vi "CalculatePhaseMagnitude_5761.vi"(7 "Max num channels":i32, 8 "unwrap phase":bool, 9 "phase reference channel":i32, 10 "previous phase":dbl[](array[numeric]), 11 "data":dbl[][](array[numeric])) -> (1 "last phase":dbl[](array[numeric]), 2 "Magnitude":dbl[][](array[numeric]), 3 "Phase":dbl[][](array[numeric]))   [LabVIEW 2018, in "Scope5782_six_channel.lvclass"]
uses:
  Scope5782_six_channel.lvclass
  <vilib>/Analysis/coordinate.llb/Angle Units.ctl
  <vilib>/Analysis/NI_AALPro.lvlib
  <vilib>/Analysis/NI_AAL_Angle.lvlib
panel:
  in  "Max num channels 2":i32
  # "each row is I and then Q of one channel"
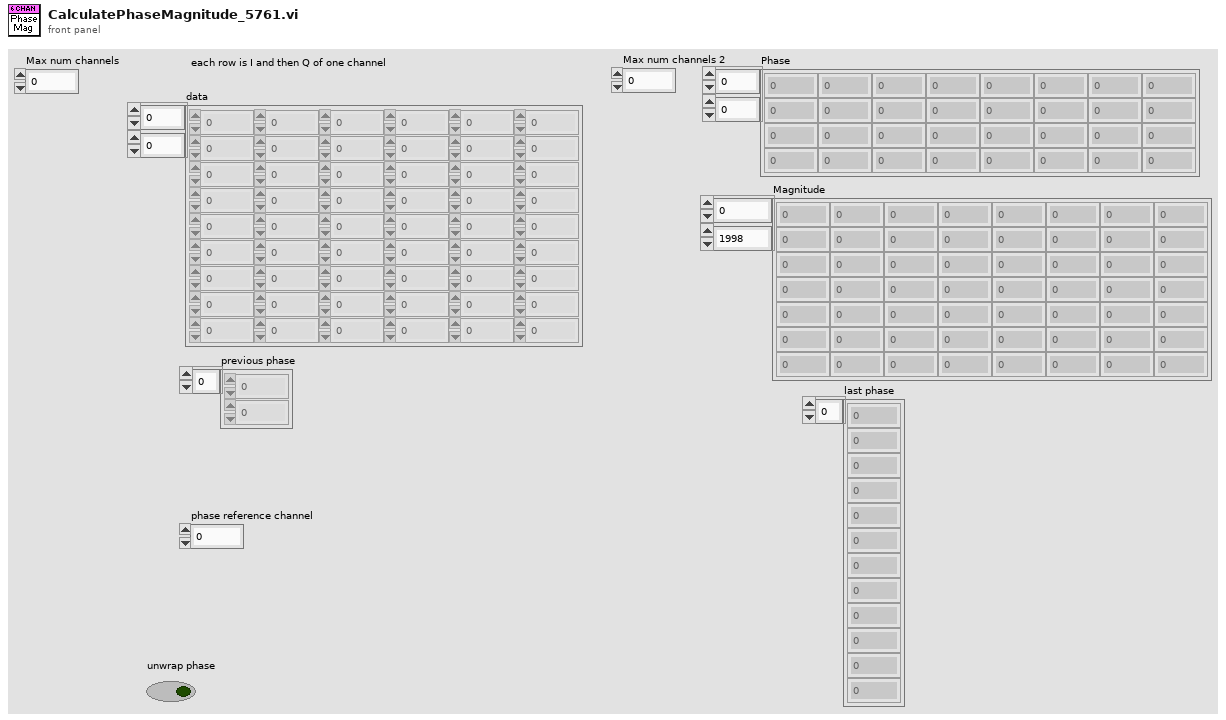
[diagram p1: front panel]
types:
  T1 = typedef "NI_AAL_Angle.lvlib/Angle Units.ctl" = i32
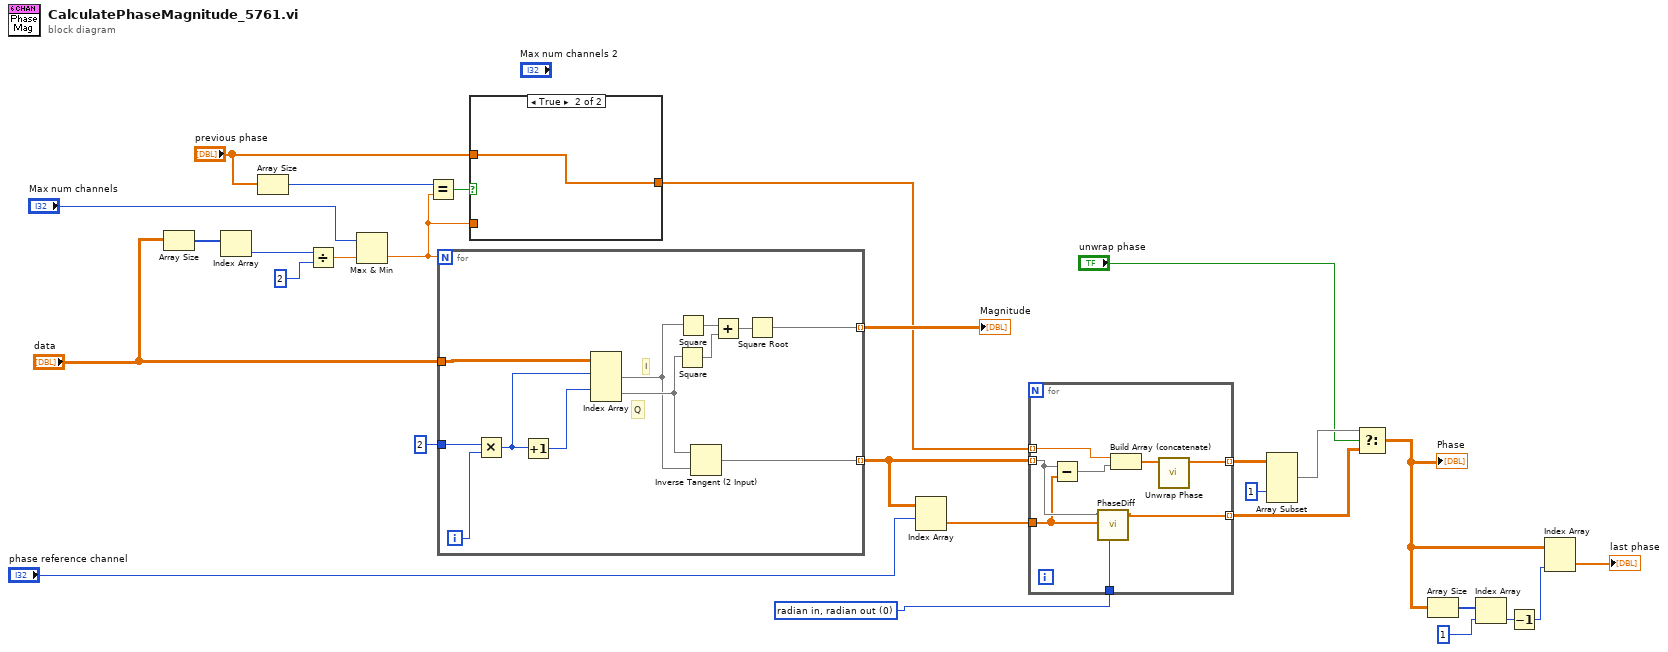
[diagram p0: block diagram]
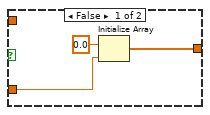
[diagram p2: hidden frame]
diagram:
  w13 = T1 0 items=["radian in, radian out", "radian in, degree out", "degree in, degree out", "degree in, radian out"] ("angle units")
  n1 = Array Size(array="data") -> (size(s)=w19:i32[])
  n2 = Index Array(array=w19) -> (element=w18:i32)  [unwired: 1 in]
  n3 = Array Size(array="previous phase") -> (size(s)=w11:i32)
  n4 = Divide(x=w18, y=2) -> (x/y=w3:dbl)
  n5 = Max & Min(x="Max num channels", y=w3) -> (min(x,y)=w2:dbl)  [unwired: 1 out]
  n6 = Equal?(x=w11, y=w2) -> (x = y?=w10:bool)
  n7 = for {
    N: w2 -> [_]
    tunnel: "data" -> [w40]
    tunnel: 2 ("y") -> [w39]
    tunnel: [w30] -> w27 mode=indexing
    tunnel: [w29] -> w12 mode=indexing
    i -> [w36]
    # "Q"
    # "I"
    n8 = Multiply(x=w39, y=w36) -> (x*y=w38:i32)
    n9 = Increment(x=w38) -> (x+1=w37:i32)
    n10 = Index Array(array=w40, index (row) #1=w38, index (row) #2=w37) -> (element #1=w31:dbl[], element #2=w32:dbl[])  [unwired: 2 in]
    n11 = Square(x=w32) -> (x^2=w34:dbl[])
    n12 = Square(x=w31) -> (x^2=w35:dbl[])
    n13 = Inverse Tangent (2 Input)(1:w31, 2:w32) -> (0:w29:dbl[])
    n14 = Add(x=w35, y=w34) -> (x+y=w33:dbl[])
    n15 = Square Root(x=w33) -> (sqrt(x)=w30:dbl[])
  }
  "Magnitude" <- w27
  n16 = case shown="True" w10 {
    tunnel: "previous phase" -> [_ w44]
    tunnel: [w41 w44] -> w8
    tunnel: w2 -> [w42 _]
    frame False {
      n17 = Initialize Array(0.0 ("element"), w42) -> (w41:dbl[])
    }
    frame True {
    }
  }
  n18 = Index Array(array=w12, index (row)="phase reference channel") -> (element=w20:dbl[])  [unwired: 1 in]
  n19 = for {
    tunnel: w12 -> [w48] mode=indexing
    tunnel: w20 -> [w47]
    tunnel: [w52] -> w14 mode=indexing
    tunnel: w8 -> [w51] mode=indexing
    tunnel: [w46] -> w5 mode=indexing
    tunnel: w13 -> [w45]
    n20 = Subtract(x=w48, y=w47) -> (x-y=w49:dbl[])
    n21 = call "PhaseDiff.vi"("angle units"=w45, "Angle 2"=w47, "Angle 1"=w48) -> ("Absolute Angle Difference"=w46:dbl[])  [unwired: 5 in]
    n22 = Build Array (concatenate)(w51, w49) -> (w50:dbl[])
    n23 = call <vilib>:"Unwrap Phase.vi"("Phase"=w50) -> ("Unwrapped Phase"=w52:dbl[])  [unwired: 9 in, 1 out]
  }
  n24 = Array Subset(array=w14, index (col)=1 ("index")) -> (w7:dbl[][])  [unwired: 3 in]
  n25 = Select(t=w7, s="unwrap phase", f=w5) -> (s? t:f=w6:dbl[][])
  "Phase" <- w6
  n26 = Array Size(array=w6) -> (size(s)=w25:i32[])
  n27 = Index Array(array=w25, index=1) -> (element=w24:i32)
  n28 = Decrement(x=w24) -> (x-1=w22:i32)
  n29 = Index Array(array=w6, index (col)=w22) -> (element=→"last phase":dbl[])  [unwired: 1 in]
